vi "Pulse Generation (Camera Link).vi"() -> ()   [LabVIEW 2023]
doc: "The Pulse Generation (Camera Link) example perfoms pulse configuration on the user-selected pulse generator. The configuration can be updated at run-time."
uses:
  <vilib>/vision/driver/NI_Vision_Acquisition_Software.lvlib
  <resource>/objmgr/imaqdx.rc
panel:
  in  "Stop":bool
  in  "Pulse Selector":string(combo)
  in  "Camera Name":refnum<k21> caption="IMAQdx Session"
  in  "Pulse Configuration":T1
  # "Overview: Demonstrates how to use the pulse capabilities of the output lines of the CameraLink Frame Grabbers.\nRequirements: Vision Acquisition Software, CameraLink Frame Grabber  \nInstructions: \n1. Select the Camera resource.\n2. Run the VI.  This will populate all of the drop down controls with the available values.\n3. Select a Pulse Selector.  This will populate the current configuration of the selected pulse generator. \n4. Configure the pulse through the Pulse Configuration settings.\n5. Select an Output Line on which the pulse is going to be generated."
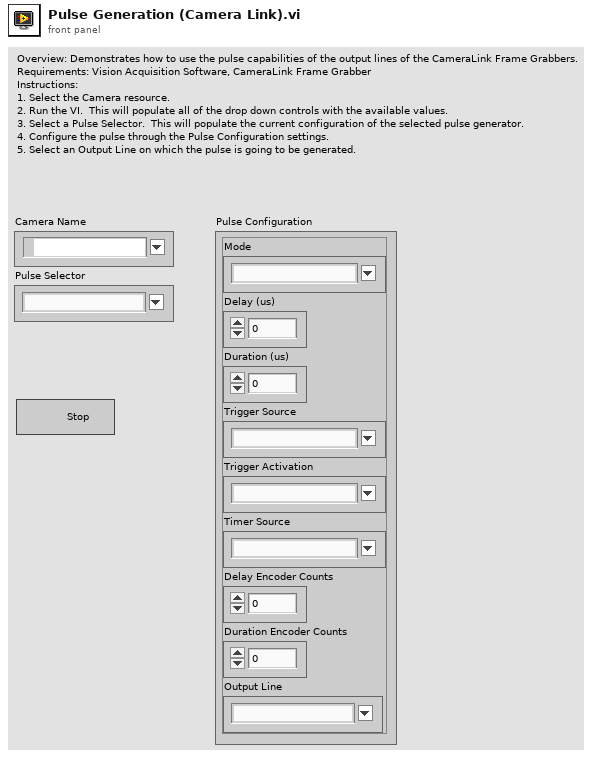
[diagram p1: front panel]
types:
  T1 = cluster{"Mode":string, "Delay (us)":dbl, "Duration (us)":dbl, "Trigger Source":string, "Trigger Activation":string, "Timer Source":string, "Delay Encoder Counts":u32, "Duration Encoder Counts":u32, "Output Line":string}
  T2 = typedef "IMAQdx.ctl" = refnum<k21>
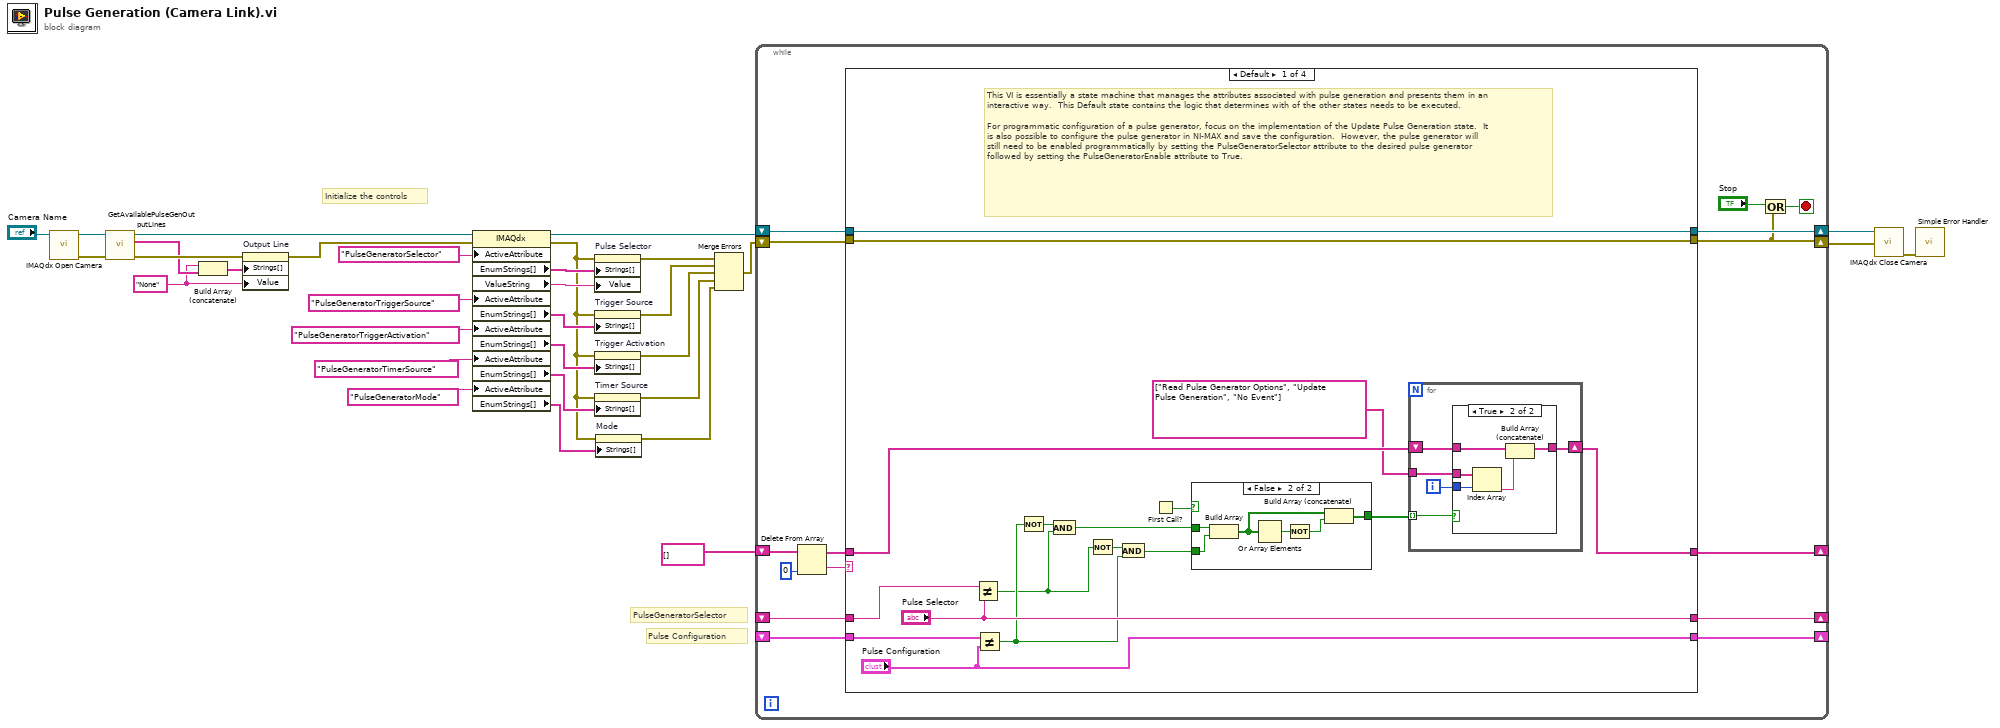
[diagram p0: block diagram]
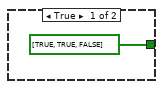
[diagram p2: hidden frame]
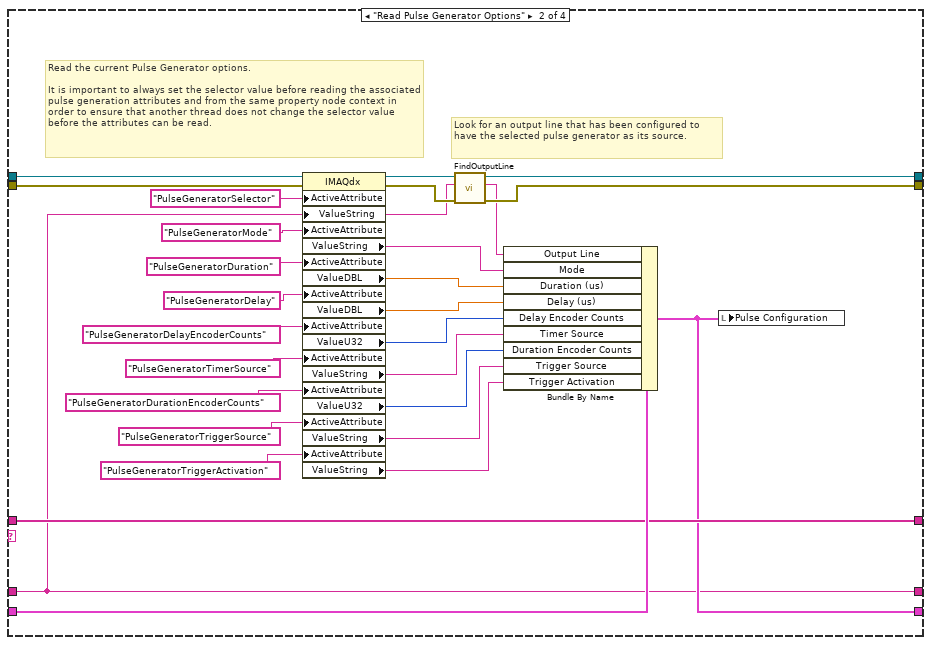
[diagram p4: hidden frame]
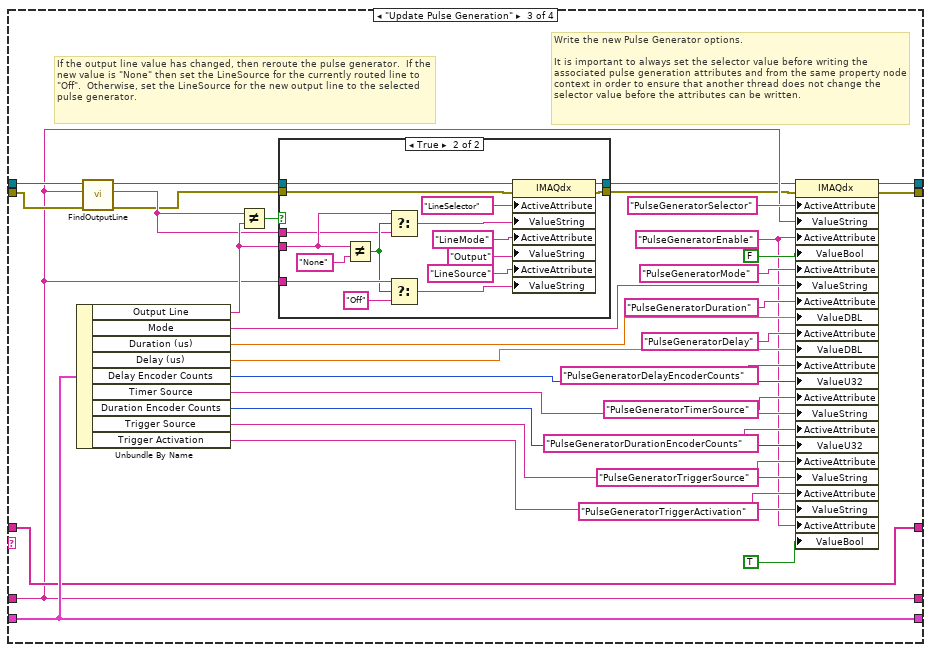
[diagram p5: hidden frame]
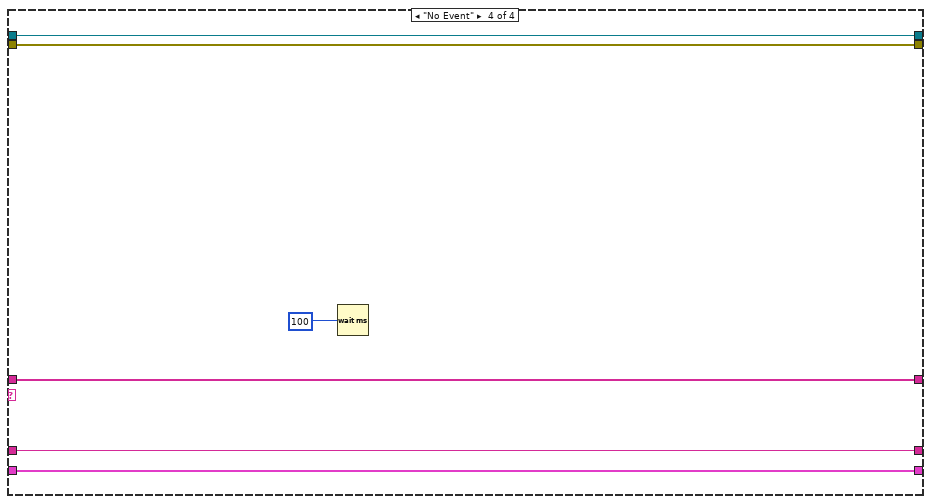
[diagram p7: hidden frame]
diagram:
  w5 = "None" ("string")
  # "Pulse Configuration"
  # "Initialize the controls"
  # "PulseGeneratorSelector"
  n1 = call <vilib>:"IMAQdx Open Camera.vi"("Session In"="Camera Name") -> ("error out"=w12:errorcluster, "Session Out"=w13:T2)  [unwired: 2 in, 7 out]
  n2 = call "GetAvailablePulseGenOutputLines.vi"("error in (no error)"=w12, "IMAQdx Session In"=w13) -> ("error out"=w11:errorcluster, "Available Output Lines"=w8:string[], "IMAQdx Session Out"=w10:T2)  [unwired: 7 in]
  n3 = Build Array (concatenate)(w5, w8) -> (w7:string[])
  n4 = property on="Output Line" class="CmbBox"(error in=w11, "Strings[]"=w7, "Value"=w5) -> (error out=w9:errorcluster)  [unwired: 1 in, 1 out]
  n5 = property class="IMAQdx"(reference=w10, error in=w9, "ActiveAttribute"="PulseGeneratorSelector", "ActiveAttribute"="PulseGeneratorTriggerSource", "ActiveAttribute"="PulseGeneratorTriggerActivation", "ActiveAttribute"="PulseGeneratorTimerSource", "ActiveAttribute"="PulseGeneratorMode") -> (reference out=w28:T2, error out=w1:errorcluster, "EnumStrings[]"=w26:string[], "ValueString"=w6:string, "EnumStrings[]"=w24:string[], "EnumStrings[]"=w22:string[], "EnumStrings[]"=w19:string[], "EnumStrings[]"=w3:string[])
  n6 = property on="Pulse Selector" class="CmbBox"(error in=w1, "Strings[]"=w26, "Value"=w6) -> (error out=w21:errorcluster)  [unwired: 1 in, 1 out]
  n7 = property on="Trigger Source" class="CmbBox"(error in=w1, "Strings[]"=w24) -> (error out=w16:errorcluster)  [unwired: 1 in, 1 out]
  n8 = property on="Trigger Activation" class="CmbBox"(error in=w1, "Strings[]"=w22) -> (error out=w15:errorcluster)  [unwired: 1 in, 1 out]
  n9 = property on="Timer Source" class="CmbBox"(error in=w1, "Strings[]"=w19) -> (error out=w14:errorcluster)  [unwired: 1 in, 1 out]
  n10 = property on="Mode" class="CmbBox"(error in=w1, "Strings[]"=w3) -> (error out=w2:errorcluster)  [unwired: 1 in, 1 out]
  n11 = Merge Errors(w21, w16, w15, w14, w2) -> (w20:errorcluster)
  n12 = while {
    shift-right: [w35] -> _
    shift-left: _ -> [w36]
    shift-right: [w45] -> _
    shift-left: _ -> [w34]
    shift-right: [w42] -> w17
    shift-left: w28 -> [w47]
    shift-right: [w41] -> w31
    shift-left: w20 -> [w46]
    shift-right: [w37] -> _
    shift-left: string[] [] -> [w39]
    stop <- w43 stop-if-true
    n13 = Delete From Array(array=w39, index=0) -> (deleted portion=w33:string, array with subset deleted=w38:string[])  [unwired: 1 in]
    n14 = case shown="Default" w33 {
      tunnel: w47 -> [w64 w92 w122 w167]
      tunnel: w46 -> [w63 w110 w121 w166]
      tunnel: [w64 w88 w144 w167] -> w42
      tunnel: [w63 w87 w128 w166] -> w41
      tunnel: ["Pulse Configuration" w90 w127 w163] -> w45
      tunnel: w38 -> [w61 w93 w126 w165]
      tunnel: [w60 w93 w126 w165] -> w37
      tunnel: w36 -> [w59 w83 w115 w164]
      tunnel: ["Pulse Selector" w83 w115 w164] -> w35
      tunnel: w34 -> [w54 w94 w127 w163]
      frame Default {
        # "This VI is essentially a state machine that manages the attributes associated with pulse generation and presents them in an interactive way.  This Default state contains the logic that determines with of the other states needs to be executed.\n\nFor programmatic configuration of a pulse generator, focus on the implementation of the Update Pulse Generation state.  It is also possible to configure the pulse generator in NI-MAX and save the configuration.  However, the pulse generator will still need to be enabled programmatically by setting the PulseGeneratorSelector attribute to the desired pulse generator followed by setting the PulseGeneratorEnable attribute to True."
        n15 = Not Equal?(x=w59, y="Pulse Selector") -> (x != y?=w48:bool)
        n16 = Not Equal?(x=w54, y="Pulse Configuration") -> (x != y?=w50:bool)
        n17 = Not(x=w50) -> (.not. x?=w49:bool)
        n18 = And(x=w49, y=w48) -> (x .and. y?=w52:bool)
        n19 = Not(x=w48) -> (.not. x?=w57:bool)
        n20 = And(x=w57, y=w50) -> (x .and. y?=w51:bool)
        n21 = First Call?() -> (First Call?: T/F=w55:bool)
        n22 = case shown="False" w55 {
          tunnel: [bool[] [TRUE, TRUE, FALSE] w69] -> w62
          tunnel: w51 -> [_ w67]
          tunnel: w52 -> [_ w66]
          frame True {
          }
          frame False {
            n23 = Build Array(w66, w67) -> (w68:bool[])
            n24 = Or Array Elements(Boolean array=w68) -> (logical OR=w70:bool)
            n25 = Not(x=w70) -> (.not. x?=w71:bool)
            n26 = Build Array (concatenate)(w68, w71) -> (w69:bool[])
          }
        }
        n27 = for {
          tunnel: w62 -> [w76] mode=indexing
          shift-right: [w74] -> w60
          shift-left: w61 -> [w75]
          tunnel: string[] ["Read Pulse Generator Options", "Update Pulse Generation", "No Event"] -> [w73]
          i -> [w72]
          n28 = case shown="True" w76 {
            tunnel: w75 -> [w77 w82]
            tunnel: w72 -> [_ w81]
            tunnel: [w77 w79] -> w74
            tunnel: w73 -> [_ w78]
            frame False {
            }
            frame True {
              n29 = Index Array(array=w78, index=w81) -> (element=w80:string)
              n30 = Build Array (concatenate)(w82, w80) -> (w79:string[])
            }
          }
        }
      }
      frame "Read Pulse Generator Options" {
        # "Look for an output line that has been configured to have the selected pulse generator as its source."
        # "Read the current Pulse Generator options.\n\nIt is important to always set the selector value before reading the associated pulse generation attributes and from the same property node context in order to ensure that another thread does not change the selector value before the attributes can be read."
        n31 = property class="IMAQdx"(reference=w92, error in=w110, "ActiveAttribute"="PulseGeneratorSelector", "ValueString"=w83, "ActiveAttribute"="PulseGeneratorMode", "ActiveAttribute"="PulseGeneratorDuration", "ActiveAttribute"="PulseGeneratorDelay", "ActiveAttribute"="PulseGeneratorDelayEncoderCounts", "ActiveAttribute"="PulseGeneratorTimerSource", "ActiveAttribute"="PulseGeneratorDurationEncoderCounts", "ActiveAttribute"="PulseGeneratorTriggerSource", "ActiveAttribute"="PulseGeneratorTriggerActivation") -> (reference out=w89:T2, error out=w86:errorcluster, "ValueString"=w102:string, "ValueDBL"=w101:dbl, "ValueDBL"=w100:dbl, "ValueU32"=w99:u32, "ValueString"=w98:string, "ValueU32"=w91:u32, "ValueString"=w97:string, "ValueString"=w96:string)
        n32 = call "FindOutputLine.vi"("error in (no error)"=w86, "Line Source"=w83, "IMAQdx Session In"=w89) -> ("error out"=w87:errorcluster, "Output Line"=w85:string, "IMAQdx Session Out"=w88:T2)  [unwired: 6 in]
        n33 = Bundle By Name(cluster=w94, "Output Line"=w85, "Mode"=w102, "Duration (us)"=w101, "Delay (us)"=w100, "Delay Encoder Counts"=w99, "Timer Source"=w98, "Duration Encoder Counts"=w91, "Trigger Source"=w97, "Trigger Activation"=w96) -> (w90:T1)
        n34 = local write "Pulse Configuration"(w90) -> ()
      }
      frame "Update Pulse Generation" {
        w117 = "PulseGeneratorEnable" ("ActiveAttribute")
        # "If the output line value has changed, then reroute the pulse generator.  If the new value is \"None\" then set the LineSource for the currently routed line to \"Off\".  Otherwise, set the LineSource for the new output line to the selected pulse generator."
        # "Write the new Pulse Generator options.\n\nIt is important to always set the selector value before writing the associated pulse generation attributes and from the same property node context in order to ensure that another thread does not change the selector value before the attributes can be written."
        n35 = Unbundle By Name(w127) -> ("Output Line"=w119:string, "Mode"=w141:string, "Duration (us)"=w139:dbl, "Delay (us)"=w137:dbl, "Delay Encoder Counts"=w125:u32, "Timer Source"=w134:string, "Duration Encoder Counts"=w124:u32, "Trigger Source"=w130:string, "Trigger Activation"=w129:string)
        n36 = call "FindOutputLine.vi"("error in (no error)"=w121, "Line Source"=w115, "IMAQdx Session In"=w122) -> ("error out"=w113:errorcluster, "Output Line"=w114:string, "IMAQdx Session Out"=w116:T2)  [unwired: 6 in]
        n37 = Not Equal?(x=w114, y=w119) -> (x != y?=w120:bool)
        n38 = case shown="True" w120 {
          tunnel: w119 -> [_ w152]
          tunnel: w116 -> [w146 w158]
          tunnel: w115 -> [_ w155]
          tunnel: w114 -> [_ w150]
          tunnel: w113 -> [w145 w149]
          tunnel: [w146 w148] -> w112
          tunnel: [w145 w147] -> w111
          frame False {
          }
          frame True {
            n39 = Not Equal?(x=w152, y="None") -> (x != y?=w153:bool)
            n40 = Select(t=w152, s=w153, f=w150) -> (s? t:f=w151:string)
            n41 = Select(t=w155, s=w153, f="Off" ("y")) -> (s? t:f=w157:string)
            n42 = property class="IMAQdx"(reference=w158, error in=w149, "ActiveAttribute"="LineSelector", "ValueString"=w151, "ActiveAttribute"="LineMode", "ValueString"="Output", "ActiveAttribute"="LineSource", "ValueString"=w157) -> (reference out=w148:T2, error out=w147:errorcluster)
          }
        }
        n43 = property class="IMAQdx"(reference=w112, error in=w111, "ActiveAttribute"="PulseGeneratorSelector", "ValueString"=w115, "ActiveAttribute"=w117, "ValueBool"=FALSE, "ActiveAttribute"="PulseGeneratorMode", "ValueString"=w141, "ActiveAttribute"="PulseGeneratorDuration", "ValueDBL"=w139, "ActiveAttribute"="PulseGeneratorDelay", "ValueDBL"=w137, "ActiveAttribute"="PulseGeneratorDelayEncoderCounts", "ValueU32"=w125, "ActiveAttribute"="PulseGeneratorTimerSource", "ValueString"=w134, "ActiveAttribute"="PulseGeneratorDurationEncoderCounts", "ValueU32"=w124, "ActiveAttribute"="PulseGeneratorTriggerSource", "ValueString"=w130, "ActiveAttribute"="PulseGeneratorTriggerActivation", "ValueString"=w129, "ActiveAttribute"=w117, "ValueBool"=TRUE) -> (reference out=w144:T2, error out=w128:errorcluster)
      }
      frame "No Event" {
        n44 = Wait (ms)(milliseconds to wait=u32 100 ("millisecond multiple")) -> ()  [unwired: 1 out]
      }
    }
    n45 = Or(x=w41, y="Stop") -> (x .or. y?=w43:bool)
  }
  n46 = call <vilib>:"IMAQdx Close Camera.vi"("error in"=w31, "Session In"=w17) -> ("error out"=w30:errorcluster)  [unwired: 9 out]
  n47 = call <vilib>:"Simple Error Handler.vi"("error in (no error)"=w30) -> ()  [unwired: 1 in, 8 out]
